vi "PalmSense Data Read Mesuarement.vi"(8 "error in (no error)":errorcluster, 9 "Message Data":variant, 11 "DMM  name":refnum<visa-resource-name>) -> (0 "error out":errorcluster, 2 "Message Data Out":variant, 3 "DMM  name out":refnum<visa-resource-name>)   [LabVIEW 2020, in "PalmSens.lvlib"]
doc: "Generates sample waveforms according to the signal type in the HW Config input."
uses:
  PalmSens.lvlib
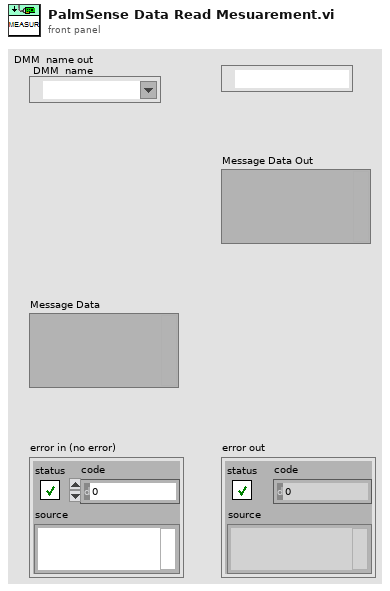
[diagram p1: front panel]
types:
  T1 = cluster{"Channel (1: Channel 1) 2":i32[], "Measurement Type":i32[]}
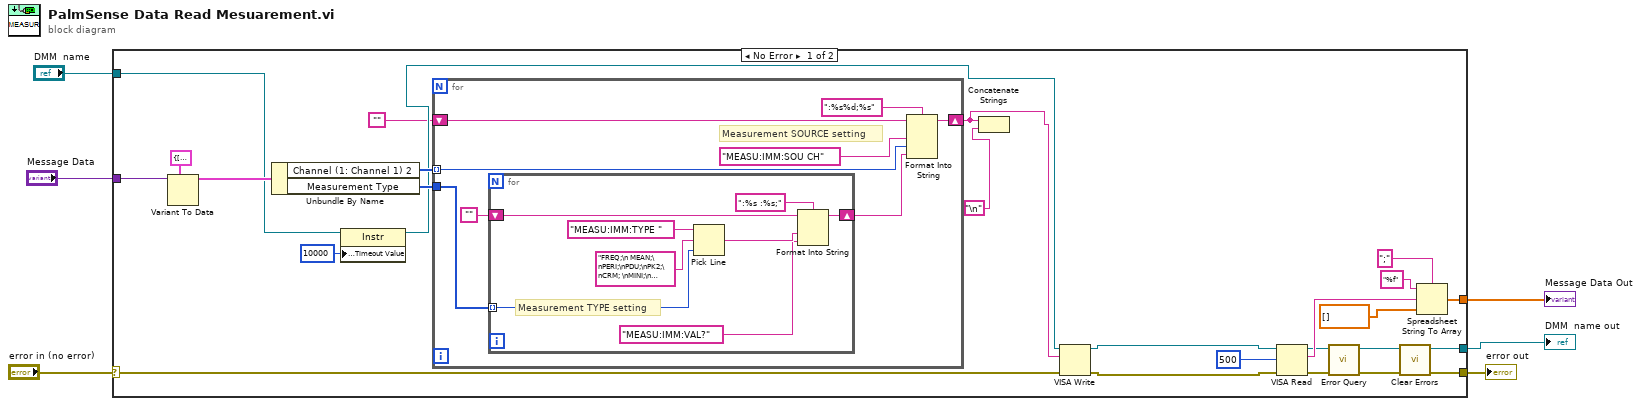
[diagram p0: block diagram]
diagram:
  n1 = case shown="No Error" "error in (no error)" {
    selector: "error in (no error)" -> [w18 w49]
    tunnel: [w7 w49] -> w5
    tunnel: "DMM  name" -> [w12 w48]
    tunnel: [w21 w48] -> w3
    tunnel: "Message Data" -> [w31 _]
    tunnel: [w20 _] -> w1
    frame No Error {
      n2 = Variant To Data(type=T1 {"Channel (1: Channel 1) 2"=[1, 2, 3], "Measurement Type"=[4, 5, 7]}, Variant=w31) -> (data=w16:T1)  [unwired: 1 in, 1 out]
      n3 = Unbundle By Name(w16) -> ("Channel (1: Channel 1) 2"=w30:i32[], "Measurement Type"=w29:i32[])
      n4 = property class="Instr"(reference=w12, "General Settings:Timeout Value"=u32 10000) -> (reference out=w11:refnum<visa-resource-name>)  [unwired: 1 in, 1 out]
      n5 = for {
        tunnel: w29 -> [w38]
        shift-right: [w32] -> w9
        shift-left: "" -> [w33]
        tunnel: w30 -> [w36] mode=indexing
        # "Measurement SOURCE setting"
        n6 = for {
          tunnel: w38 -> [w45] mode=indexing
          shift-right: [w44] -> w35
          shift-left: "" -> [w43]
          # "Measurement TYPE setting"
          n7 = Pick Line(string ("")="MEASU:IMM:TYPE ", multi-line string="FREQ;\n MEAN;\nPERI;\nPDU;\nPK2;\nCRM; \nMINI;\n MAXI;\n RIS;\nFALL;\nPWI;\nNWI;\nAMP;\nCMEAN;\nHIG;\nLOW;\nNDU;\nPOVER;\nNOVER;\nCURSORM;\nBURSTWID;\nPPULSEC;\nNPULSEC;\nREDGEC;\nFEDGEC;\nAREA;\nCAREA;\nRMS;\nCURSORR;", line index=w45) -> (output string=w41:string)
          n8 = Format Into String(format string=":%s :%s;", initial string=w43, w41, "MEASU:IMM:VAL?" ("write buffer")) -> (resulting string=w44:string)  [unwired: 1 in, 1 out]
        }
        n9 = Format Into String(format string=":%s%d;%s", initial string=w33, "MEASU:IMM:SOU CH" ("string (\"\")"), w36, w35) -> (resulting string=w32:string)  [unwired: 1 in, 1 out]
      }
      n10 = Concatenate Strings(w9, "\n") -> ()  [unwired: 1 out]
      n11 = VISA Write(VISA resource name=w11, write buffer=w9, error in (no error)=w18) -> (VISA resource name out=w28:refnum<visa-resource-name>, error out=w15:errorcluster)  [unwired: 1 out]
      n12 = VISA Read(VISA resource name=w28, byte count=u32 500, error in (no error)=w15) -> (VISA resource name out=w23:refnum<visa-resource-name>, read buffer=w26:string, error out=w22:errorcluster)  [unwired: 1 out]
      n13 = call <instrlib>:"Error Query.vi"("error in (no error)"=w22, "VISA resource name"=w23) -> ("error out"=w19:errorcluster, "VISA resource name out"=w21:refnum<visa-resource-name>)  [unwired: 8 out]
      n14 = call <vilib>:"Clear Errors.vi"("error in (no error)"=w19) -> ("error out"=w7:errorcluster)  [unwired: 5 in, 1 out]
      n15 = Spreadsheet String To Array(delimiter (Tab)=";", format string="%f" ("spreadsheet string"), spreadsheet string=w26, array type (2D Dbl)=dbl[] []) -> (array=w20:dbl[])
    }
    frame Error {
    }
  }
  "error out" <- w5
  "Message Data Out" <- w1
  "DMM  name out" <- w3
